vi "CleanUp.JUnitXML.vi"(8 "error in (no error)":errorcluster, 11 "TextTestRunner in":refnum<class "TextTestRunner.JUnitXML.lvclass">) -> (0 "error out":errorcluster, 3 "TextTestRunner out":refnum<class "TextTestRunner.JUnitXML.lvclass">)   [LabVIEW 2018, in "TextTestRunner.JUnitXML.lvclass"]
uses:
  TextTestRunner.JUnitXML.lvclass
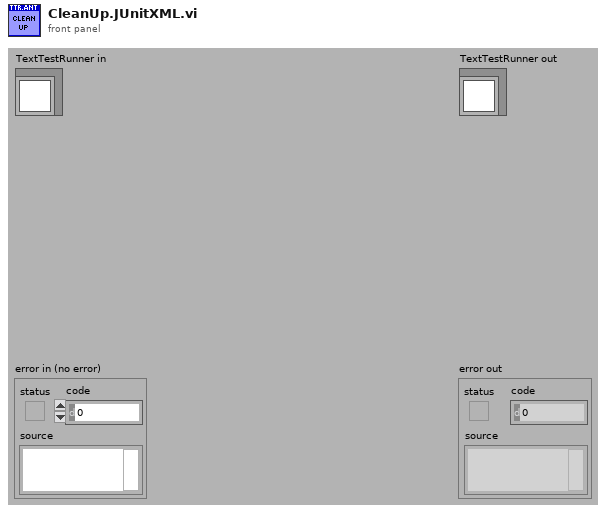
[diagram p1: front panel]
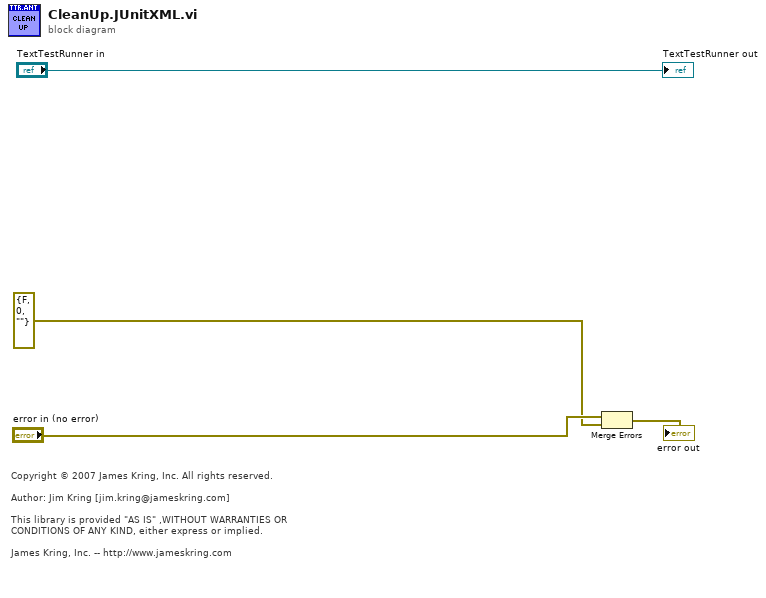
[diagram p0: block diagram]
diagram:
  # "Copyright © 2007 James Kring, Inc. All rights reserved.\n\nAuthor: Jim Kring [jim.kring@jameskring.com]\n\nThis library is provided \"AS IS\" ,WITHOUT WARRANTIES OR \nCONDITIONS OF ANY KIND, either express or implied.\n\nJames Kring, Inc. -- http://www.jameskring.com"
  n1 = Merge Errors("error in (no error)", errorcluster {"status"=FALSE, "code"=0, "source"=""} ("error in (no error)")) -> (→"error out":errorcluster)
  "TextTestRunner out" <- "TextTestRunner in"
